vi "Adam_Ch_Input_Output.vi"(4 "Simulate":bool, 5 "Duty No":u16 format="%.0b", 6 "Value to Output":dbl format="%.2f", 7 "Previuos Scan Value":dbl format="%.2f", 8 "Ch values":dbl[](array[numeric]) format="%.2f", 9 "Scan Period":dbl format="%.2f", 10 "Ch Discription":T1={"Ch Name"="", "Type"=enum."Test", "Function"=enum."Analogue Input", "Ch State"=enum."On", "Calibration type"=enum."Raw", "A"=0.0, "B"=0.0, "C"=0.0, "D"=0.0, "Comments"="", "Address"={"Main"=0, "Ch."=0, "Sub"=0, "Port Name"=""}, "String"="", "Duty"=65535} {"Duty" format="%.0b"; "D" format="%#_5g"; "C" format="%#_5g"; "B" format="%#_5g"; "A" format="%#_5g"}, 11 "Ch names":string[](array[string])) -> (0 "Scan comment":string, 3 "Calibrated units":dbl format="%.2f")   [LabVIEW 2010]
uses:
  ADAM Client/Sub VIs/ADAM Controls/Ch_description_ADAM.ctl
  ADAM Client/Sub VIs/ADAM Controls/Module_type_ADAM.ctl
  ADAM Client/Sub VIs/ADAM Controls/Function_ADAM.ctl
  ADAM Client/Sub VIs/ADAM Controls/Channel_State.ctl
  ADAM Client/Sub VIs/ADAM Controls/Calib_type_ADAM.ctl
  ADAM Client/Sub VIs/ADAM Controls/Address.ctl
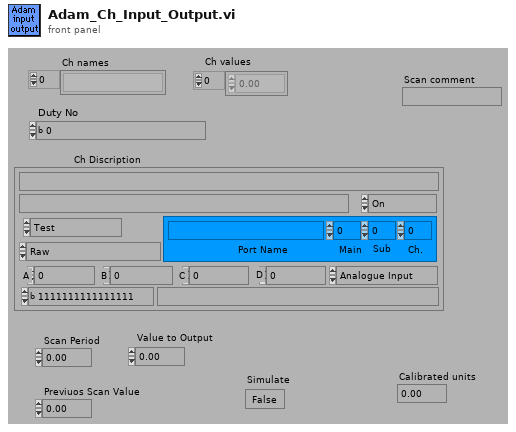
[diagram p1: front panel]
types:
  T1 = typedef "Ch_description_ADAM.ctl" = cluster{"Ch Name":string, "Type":T2, "Function":T3, "Ch State":T4, "Calibration type":T5, "A":dbl, "B":dbl, "C":dbl, "D":dbl, "Comments":string, "Address":T6, "String":string, "Duty":u16}
  T2 = typedef "Module_type_ADAM.ctl" = enum16{"4011", "4012", "4013", "4014", "4016", "4017", "4018", "4021", "4050", "4052", "4053", "4060", "4080", "5000", "5017", "5018", "5024", "5051", "5056", "5060", "6060", "Tracker", "WEST", "GILL", "JEM", "VICI", "Vaisala", "DRUCK", "Run VI Named:", "IR2100", "PPT", "Comparator", "VIRTUAL", "Hold Value", "Read A", "Read Ch", "Coded", "Client Info", "Web Client", "X10", "Test"}
  T3 = typedef "Function_ADAM.ctl" = enum16{"Analogue Input", "Digital Input", "Event counter", "Event rate", "Analogue Output", "Digital Output", "Relay Output"}
  T4 = typedef "Channel_State.ctl" = enum16{"On", "Off", "Always On", "Always Off"}
  T5 = typedef "Calib_type_ADAM.ctl" = enum16{"Raw", "Bx + A", "Cx^2 + Bx + A", "Dx^3 + Cx^2 + Bx + A", "In Band", "Hi-Tec Q", "Hi-Tec M_dot", "Text"}
  T6 = typedef "Address.ctl" = cluster{"Main":i32, "Ch.":i32, "Sub":i32, "Port Name":string}
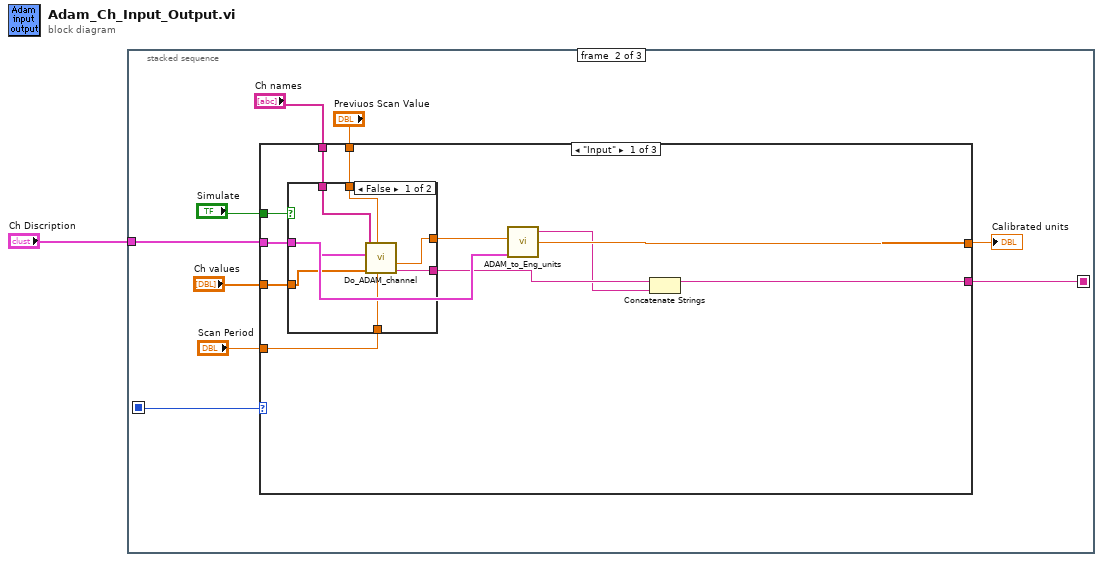
[diagram p0: block diagram]
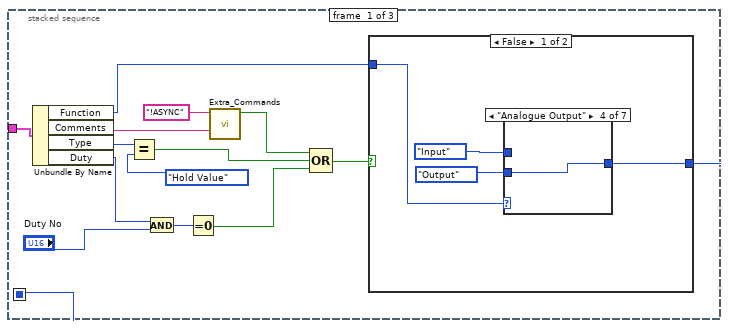
[diagram p2: hidden frame]
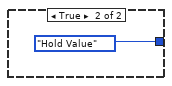
[diagram p9: hidden frame]
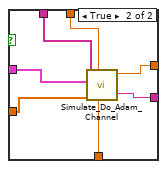
[diagram p10: hidden frame]
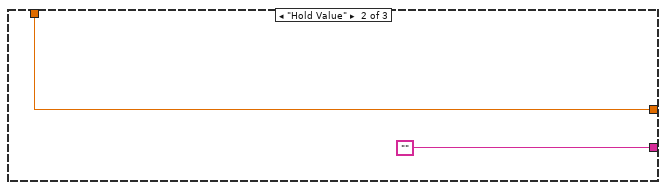
[diagram p11: hidden frame]
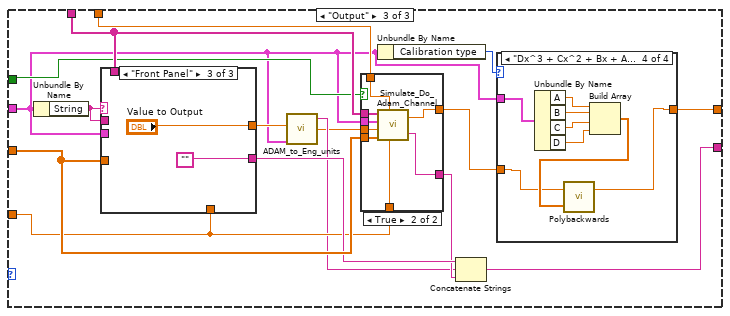
[diagram p12: hidden frame]
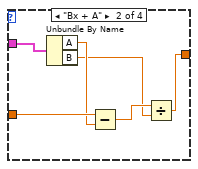
[diagram p14: hidden frame]
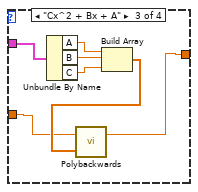
[diagram p15: hidden frame]
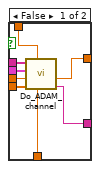
[diagram p16: hidden frame]
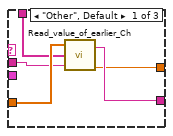
[diagram p17: hidden frame]
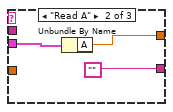
[diagram p18: hidden frame]
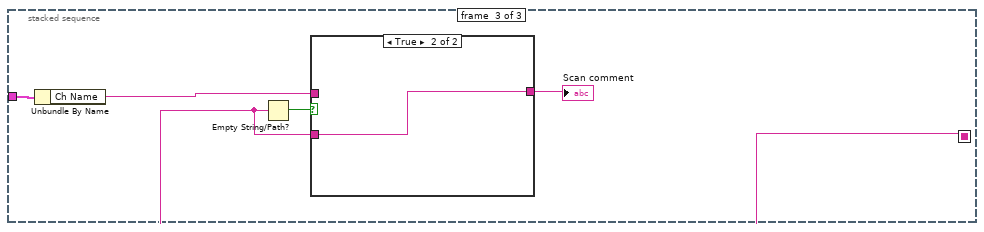
[diagram p19: hidden frame]
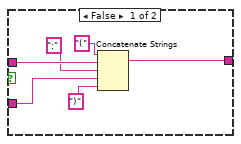
[diagram p20: hidden frame]
diagram:
  n1 = stacked-sequence {
    seq-local: [w10 _ _] -> [_ w31 _]
    seq-local: [_ w30 _] -> [_ _ w128]
    tunnel: "Ch Discription" -> [w15 w33 w130]
    frame #0 {
      n2 = Unbundle By Name(w15) -> ("Function"=w11:T3, "Comments"=w8:string, "Type"=w14:T2, "Duty"=w6:u16)
      n3 = Equal?(x=w14, y=Module_type_ADAM."Hold Value" ("Type")) -> (x = y?=w12:bool)
      n4 = And(x=w6, y="Duty No") -> (x .and. y?=w4:u16)
      n5 = Equal To 0?(x=w4) -> (x = 0?=w3:bool)
      n6 = call "Extra_Commands.vi"("String to Search"=w8, "Command"="!ASYNC" ("String to match")) -> ("Command Found"=w7:bool)  [unwired: 1 in, 4 out]
      n7 = Compound Arithmetic op=OR(w7, w12, w3) -> (w2:bool)
      n8 = case shown="False" w2 {
        tunnel: w11 -> [w17 _]
        tunnel: [w16 enum16{"Input", "Output", "Hold Value"}."Hold Value"] -> w10
        frame False {
          n9 = case shown="\"Analogue Output\"" w17 {
            tunnel: [w20 w21 w22 w23 w24 w25 w26] -> w16
            tunnel: enum16{"Input", "Output", "Hold Value"}."Input" -> [w20 w21 w22 _ _ _ w26]
            tunnel: enum16{"Input", "Output", "Hold Value"}."Output" -> [_ _ _ w23 w24 w25 _]
            frame "Analogue Input" {
            }
            frame "Event counter" {
            }
            frame "Event rate" {
            }
            frame "Analogue Output" {
            }
            frame "Digital Output" {
            }
            frame "Relay Output" {
            }
            frame "Digital Input" {
            }
          }
        }
        frame True {
        }
      }
    }
    frame #1 {
      n10 = case shown="\"Input\"" w31 {
        tunnel: [w47 w63 w66] -> w36
        tunnel: "Scan Period" -> [w42 _ w71]
        tunnel: "Ch values" -> [w45 _ w79]
        tunnel: "Ch names" -> [w44 _ w78]
        tunnel: [w38 "" w77] -> w30
        tunnel: w33 -> [w43 _ w64]
        tunnel: "Previuos Scan Value" -> [w41 w63 w75]
        tunnel: "Simulate" -> [w37 _ w68]
        frame "Input" {
          n11 = case shown="False" w37 {
            tunnel: [w54 w61] -> w46
            tunnel: w45 -> [w53 w60]
            tunnel: w44 -> [w52 w59]
            tunnel: w43 -> [w51 w58]
            tunnel: w42 -> [w50 w57]
            tunnel: w41 -> [w49 w56]
            tunnel: [w48 w55] -> w40
            frame False {
              n12 = call "Do_ADAM_channel.vi"("Scan Period"=w50, "Previous Scan Value"=w49, "Present scan array"=w53, "Ch Description"=w51, "Ch names"=w52) -> ("Scan comment"=w48:string, "Output"=w54:dbl)  [unwired: 1 in, 2 out]
            }
            frame True {
              n13 = call "Simulate_Do_Adam_Channel.vi"("Scan Period"=w57, "Previuos Scan Value"=w56, "Ch values"=w60, "Ch Discription"=w58, "Ch names"=w59) -> ("Scan comment"=w55:string, "Calibrated units"=w61:dbl)  [unwired: 1 in]
            }
          }
          n14 = call "ADAM_to_Eng_units.vi"("Ch Description"=w43, "Raw"=w46) -> ("Calibrated units"=w47:dbl, "Comments"=w39:string)  [unwired: 1 in, 2 out]
          n15 = Concatenate Strings(w40, w39) -> (w38:string)
        }
        frame "Hold Value" {
        }
        frame "Output" {
          n16 = Unbundle By Name(w64) -> ("String"=w74:string)
          n17 = case shown="\"Front Panel\"" w74 {
            tunnel: w64 -> [_ w125 _]
            tunnel: w79 -> [w122 _ _]
            tunnel: w78 -> [w121 _ _]
            tunnel: w74 -> [w120 _ _]
            tunnel: [w119 "" ""] -> w76
            tunnel: w71 -> [_ _ _]
            tunnel: [w118 w123 "Value to Output"] -> w72
            frame "Other", Default {
              n18 = call "Read_value_of_earlier_Ch.vi"("Desired Ch to Read"=w120, "Ch names"=w121, "Present scan array"=w122) -> ("Value"=w118:dbl, "Scan comment"=w119:string)  [unwired: 1 in]
            }
            frame "Read A" {
              n19 = Unbundle By Name(w125) -> ("A"=w123:dbl)
            }
            frame "Front Panel" {
            }
          }
          n20 = call "ADAM_to_Eng_units.vi"("Ch Description"=w64, "Raw"=w72) -> ("Calibrated units"=w69:dbl, "Comments"=w70:string)  [unwired: 1 in, 2 out]
          n21 = case shown="True" w68 {
            tunnel: w79 -> [w109 w117]
            tunnel: w78 -> [w108 w116]
            tunnel: [w107 w115] -> w65
            tunnel: w75 -> [w106 w114]
            tunnel: [w105 w113] -> w73
            tunnel: w71 -> [w104 w112]
            tunnel: w64 -> [w103 w111]
            tunnel: w69 -> [w102 w110]
            frame False {
              n22 = call "Do_ADAM_channel.vi"("Scan Period"=w104, "Previous Scan Value"=w106, "Present scan array"=w109, "Value to Output"=w102, "Ch Description"=w103, "Ch names"=w108) -> ("Scan comment"=w105:string, "Output"=w107:dbl)  [unwired: 2 out]
            }
            frame True {
              n23 = call "Simulate_Do_Adam_Channel.vi"("Scan Period"=w112, "Previuos Scan Value"=w114, "Ch values"=w117, "Value to Output"=w110, "Ch Discription"=w111, "Ch names"=w116) -> ("Scan comment"=w113:string, "Calibrated units"=w115:dbl)
            }
          }
          n24 = Unbundle By Name(w64) -> ("Calibration type"=w67:T5)
          n25 = Concatenate Strings(w76, w70, w73) -> (w77:string)
          n26 = case shown="\"Dx^3 + Cx^2 + Bx + A\"" w67 {
            tunnel: [w80 w81 w87 w95] -> w66
            tunnel: w65 -> [w80 w85 w88 w96]
            tunnel: w64 -> [_ w86 w93 w101]
            frame "Raw", Default {
            }
            frame "Bx + A" {
              n27 = Unbundle By Name(w86) -> ("A"=w84:dbl, "B"=w82:dbl)
              n28 = Subtract(x=w85, y=w84) -> (x-y=w83:dbl)
              n29 = Divide(x=w83, y=w82) -> (x/y=w81:dbl)
            }
            frame "Cx^2 + Bx + A" {
              n30 = Unbundle By Name(w93) -> ("A"=w92:dbl, "B"=w91:dbl, "C"=w90:dbl)
              n31 = Build Array(w92, w91, w90) -> (w89:dbl[])
              n32 = call "Polybackwards.vi"("Coefficients"=w89, "Y input"=w88) -> ("X output"=w87:dbl)  [unwired: 1 out]
            }
            frame "Dx^3 + Cx^2 + Bx + A" {
              n33 = Unbundle By Name(w101) -> ("A"=w100:dbl, "B"=w99:dbl, "C"=w98:dbl, "D"=w94:dbl)
              n34 = Build Array(w100, w99, w98, w94) -> (w97:dbl[])
              n35 = call "Polybackwards.vi"("Coefficients"=w97, "Y input"=w96) -> ("X output"=w95:dbl)  [unwired: 1 out]
            }
          }
        }
      }
      "Calibrated units" <- w36
    }
    frame #2 {
      n36 = Unbundle By Name(w130) -> ("Ch Name"=w129:string)
      n37 = Empty String/Path?(string/path=w128) -> (empty?=w131:bool)
      n38 = case shown="True" w131 {
        tunnel: w129 -> [w137 _]
        tunnel: w128 -> [w135 w139]
        tunnel: [w133 w139] -> w132
        frame False {
          n39 = Concatenate Strings("(", w137, ":" ("Scan comment"), w135, ")") -> (w133:string)
        }
        frame True {
        }
      }
      "Scan comment" <- w132
    }
  }
